vi "MAIN_merFISH_open_close_valve.vi"(0 "Log file":refnum<file>, 1 "Hybridization procedure not empty?":bool, 2 "queue piezo":refnum<queue>, 3 "queue ASI stage":refnum<queue>, 4 "queue valve":refnum<queue>, 5 "Starting time":dbl, 7 "Measure QPD":bool caption="Calibration", 9 "variant":variant, 11 "error in":errorcluster, 12 "Two-way valve":refnum<vi>) -> (6 "Next task":T1, 15 "error out":errorcluster)   [LabVIEW 2015]
uses:
  CONTROLS/Q_ASI_stage_element.ctl
  CONTROLS/Q_MCL_piezo_element.ctl
  CONTROLS/Q_main_element.ctl
  CONTROLS/Q_VALVE_element.ctl
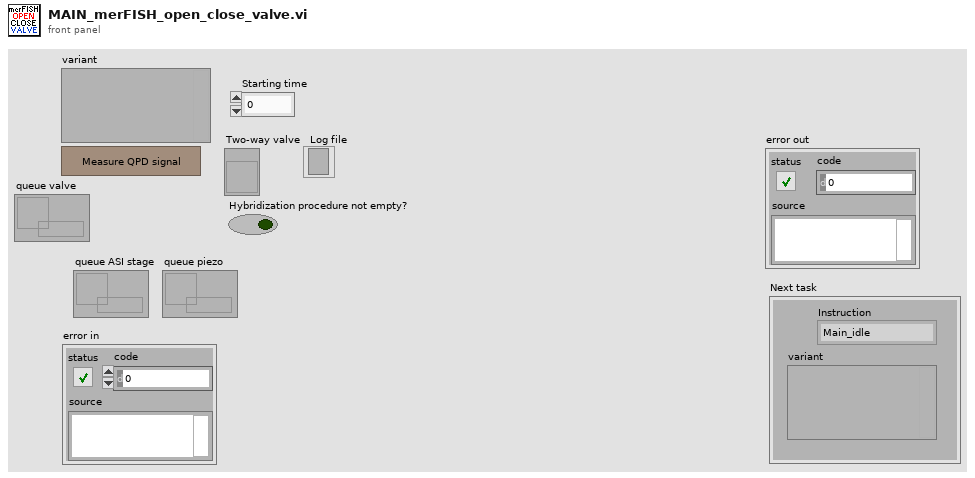
[diagram p1: front panel]
types:
  T1 = typedef "Q_main_element.ctl" = cluster{"variant":variant, "Instruction":enum16{"Main_idle", "Main_initialize", "Main_initialize_TDMS", "Main_initialize_Queue", "Main_error", "Main_DAQ_initialization_results", "Main_ASI_initialization_results", "Main_Piezo_initialization_results", "Main_Valve_initialization_results", "Main_Pump_initialization_results", "Main_CAMERA_initialization_results", "Main_FPGA_initialization_results", "Main_DAQ_error", "Main_ASI_error", "Main_Piezo_error", "Main_CAMERA_error", "Main_Valve_error", "Main_Pump_error", "Main_FPGA_error", "Main_start_acquiring", "Main_not_acquiring", "Main_acquiring", "Main_stop_acquiring", "Main_change_exposure", "Main_change_z_scan_parameters", "Main_define_ROI", "Main_define_mosaic", "Main_read_kinetic_time", "Main_cooler", "Main_read_temperature", "Main_save_XY", "Main_load_XY", "Main_discard_XY", "Main_move_to_XY", "Main_measure_QPD", "Main_autofocus_calibration", "Main_autofocus_initialization", "Main_autofocus_stop", "Main_save_PID", "Main_change_H_valve_position", "Main_two_way_valve", "Main_save_movie", "Main_init_single_scan", "Main_single_scan", "Main_stop_single_scan", "Main_merFISH_illumination_parameters", "Main_merFISH_buffer_probe_list", "Main_merFISH_injections_procedure", "Main_merFISH_save_setpoint", "Main_merFISH_DAPI_parameters", "Main_merFISH_Brightfield_parameters", "Main_merFISH_save_embryo_ROI", "Main_merFISH_init", "Main_merFISH_resume", "Main_merFISH_start_autofocus", "Main_merFISH_open_close_valve_merFISH", "Main_merFISH_open_close_valve_photobleaching", "Main_merFISH_hybridization", "Main_merFISH_move_to_ROI", "Main_merFISH_wait_stabilization", "Main_merFISH_move_to_REF", "Main_merFISH_scan", "Main_merFISH_photobleaching_injection", "Main_merFISH_photobleaching", "Main_merFISH_send_email", "Main_merFISH_close", "Main_STOP"}}
  T2 = typedef "Q_MCL_piezo_element.ctl" = cluster{"variant":variant, "Instruction":enum16{"Piezo_idle", "Piezo_initialize", "Piezo_error", "Piezo_security_stop", "Piezo_read_z", "Piezo_move_z", "Piezo_keyboard_move", "Piezo_close_autofocus_calibration_ramp", "Piezo_change_init_state", "Piezo_init_autofocus", "Piezo_init_autofocus_merFISH_TL", "Piezo_autofocus", "Piezo_autofocus_merFISH_TL", "Piezo_stop_autofocus", "Piezo_stop_autofocus_merFISH_TL", "Piezo_autofocus_lost", "Piezo_resume_autofocus_merFISH_TL", "Piezo_check_z_position_merFISH_TL", "Piezo_init_ramp", "Piezo_move_z_ramp", "Piezo_close_ramp", "Piezo_close_merFISH", "Piezo_stop"}}
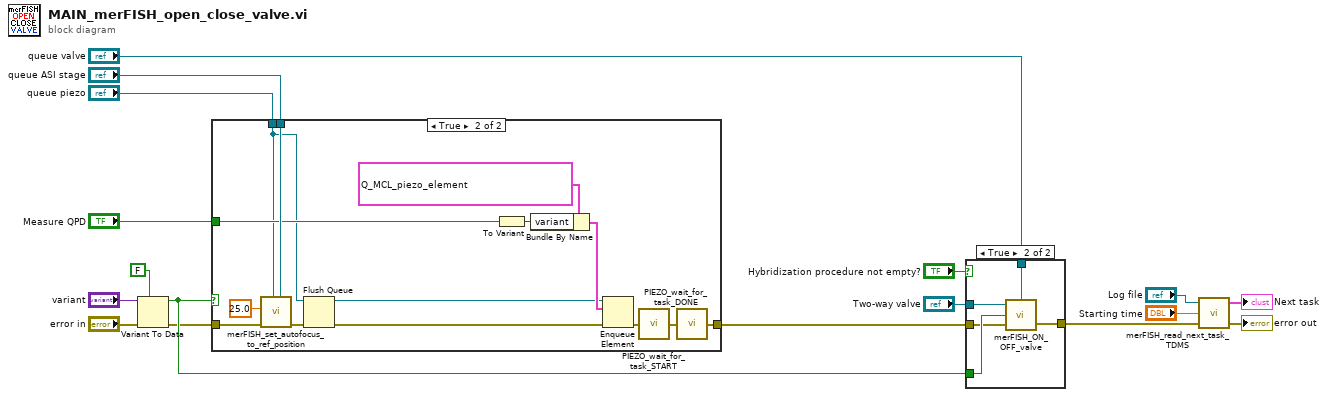
[diagram p0: block diagram]
diagram:
  n1 = Variant To Data(error in="error in", type=FALSE, Variant="variant") -> (data=w17:bool, error out=w15:errorcluster)
  n2 = case shown="True" w17 {
    tunnel: w15 -> [w18 w32]
    tunnel: "queue ASI stage" -> [_ w31]
    tunnel: "Measure QPD" -> [_ w29]
    tunnel: [w18 w21] -> w16
    tunnel: "queue piezo" -> [_ w20]
    frame False {
    }
    frame True {
      n3 = call "merFISH_set_autofocus_to_ref_position.vi"("queue ASI stage"=w31, "queue piezo"=w20, "error in"=w32, "Ref"=25.0) -> ("error out"=w30:errorcluster)  [unwired: 7 in]
      n4 = Flush Queue(queue=w20, error in (no error)=w30) -> (queue out=w25:refnum<queue>, error out=w24:errorcluster)  [unwired: 1 out]
      n5 = To Variant(anything=w29) -> (Variant=w27:variant)
      n6 = Bundle By Name(cluster=T2 {"variant"=variant, "Instruction"=enum."Piezo_stop_autofocus_merFISH_TL"} ("element"), "variant"=w27) -> (w28:T2)
      n7 = Enqueue Element(queue=w25, element=w28, error in (no error)=w24) -> (error out=w23:errorcluster)  [unwired: 1 in, 2 out]
      n8 = call "PIEZO_wait_for_task_START.vi"("error in"=w23) -> ("error out"=w22:errorcluster)
      n9 = call "PIEZO_wait_for_task_DONE.vi"("error in"=w22) -> ("error out"=w21:errorcluster)
    }
  }
  n10 = case shown="True" "Hybridization procedure not empty?" {
    tunnel: "queue valve" -> [_ w35]
    tunnel: [w33 w34] -> w13
    tunnel: w17 -> [_ w38]
    tunnel: w16 -> [w33 w37]
    tunnel: "Two-way valve" -> [_ w36]
    frame False {
    }
    frame True {
      n11 = call "merFISH_ON_OFF_valve.vi"("queue valve"=w35, "error in"=w37, "Valve on off"=w38, "Two-way Refnum"=w36) -> ("error out"=w34:errorcluster)  [unwired: 1 in]
    }
  }
  n12 = call "merFISH_read_next_task_TDMS.vi"("error in"=w13, "Starting time"="Starting time", "Log file"="Log file") -> ("error out"=→"error out":errorcluster, "task"=→"Next task":T1)  [unwired: 1 in]
